vi "FS Sketch Line.vi"(8 "Sketch #":i32=1, 9 "Line":T2={"Pt1 x"=0.0, "Pt1 y"=0.0, "Pt2 x"=2.0, "Pt2 y"=4.0}, 10 "Sketch Plane":T1, 11 "Feature In":string="FeatureScript 1247;\nimport(path : \"onshape/std/geometry.fs\", version : \"1247.0\");\n\nannotation { \"Feature Type Name\" : \"LabVIEW Feature\" }\nexport const myFeature = defineFeature(function(context is Context, id is Id, definition is map)\n    precondition\n    {\n        // Define the parameters of the feature type\n    }\n    {\n        // Define the function's action\n    });") -> (3 "Feature Out":string="FeatureScript 1247;\nimport(path : \"onshape/std/geometry.fs\", version : \"1247.0\");\n\nannotation { \"Feature Type Name\" : \"LVFeat1\" }\nexport const myFeature = defineFeature(function(context is Context, id is Id, definition is map)\n    precondition\n    {\n        // Define the parameters of the feature type\n    }\n    {\n        // Define the function's action\n\nvar sketch1 = newSketch(context, id + \"sketch1\", {\n                \"sketchPlane\" : qCreatedBy(makeId(\"Top\"), EntityType.FACE)\n        });\n        // Create sketch entities here\n        skRectangle(sketch1, \"rectangle1\", {\n                \"firstCorner\" : vector(0, 0) * inch,\n                \"secondCorner\" : vector(3, 4) * inch\n        });\n        \n        skSolve(sketch1);\n    });")   [LabVIEW 2019]
uses:
  Users/matt/Documents/LabVIEW/Sketch Plane.ctl
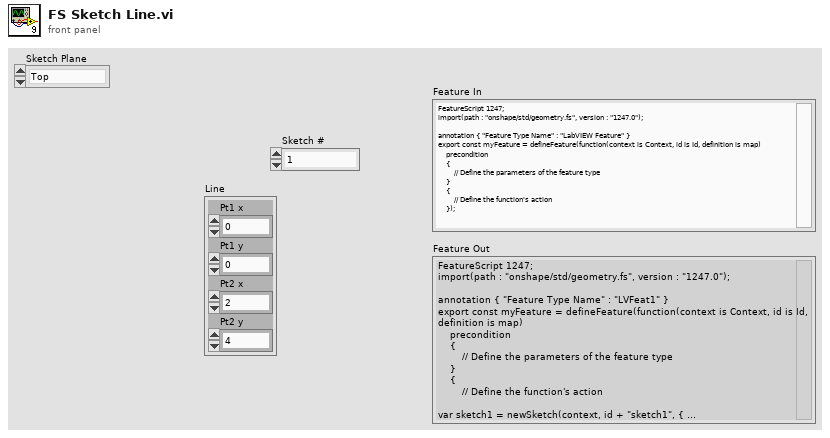
[diagram p1: front panel]
types:
  T1 = typedef "Sketch Plane.ctl" = enum16{"Top", "Front", "Right", "plane1", "plane2", "plane3"}
  T2 = cluster{"Pt1 x":dbl, "Pt1 y":dbl, "Pt2 x":dbl, "Pt2 y":dbl}
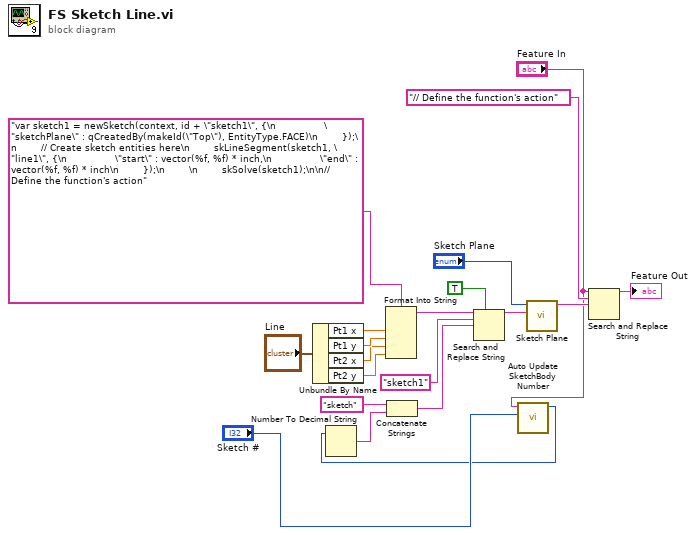
[diagram p0: block diagram]
diagram:
  n1 = Unbundle By Name("Line") -> ("Pt1 x"=w9:dbl, "Pt1 y"=w8:dbl, "Pt2 x"=w7:dbl, "Pt2 y"=w6:dbl)
  n2 = Format Into String(format string="var sketch1 = newSketch(context, id + \"sketch1\", {\n                \"sketchPlane\" : qCreatedBy(makeId(\"Top\"), EntityType.FACE)\n        });\n        // Create sketch entities here\n        skLineSegment(sketch1, \"line1\", {\n                \"start\" : vector(%f, %f) * inch,\n                \"end\" : vector(%f, %f) * inch\n        });\n        \n        skSolve(sketch1);\n\n// Define the function's action" ("string"), w9, w8, w7, w6) -> (resulting string=w5:string)  [unwired: 2 in, 1 out]
  n3 = call <userlib>:"Auto Update SketchBody Number.vi"("Sketch # in"="Sketch #", "Feature In"="Feature In") -> ("Sketch # out"=w1:i32)  [unwired: 8 in, 1 out]
  n4 = Number To Decimal String(number=w1) -> (decimal integer string=w13:string)  [unwired: 1 in]
  n5 = Concatenate Strings("sketch" ("regular expression"), w13) -> (w14:string)
  n6 = Search and Replace String(replace all?=TRUE ("replace all? (F)"), input string=w5, search string="sketch1" ("regular expression"), replace string=w14) -> (result string=w12:string)  [unwired: 4 in, 3 out]
  n7 = call <userlib>:"Sketch Plane.vi"("result string in"=w12, "Sketch Plane"="Sketch Plane") -> ("result string out"=w11:string)  [unwired: 9 in]
  n8 = Search and Replace String(input string="Feature In", search string="// Define the function's action", replace string=w11) -> (result string=→"Feature Out":string)  [unwired: 5 in, 3 out]
